vi "Add Message Handler.vi"(8 "error in (no error)":errorcluster, 10 "TCPMessageHandler":refnum<class "TCPMessageHandler.lvclass">, 11 "TCPMessaging in":refnum<class "TCPMessaging.lvclass">) -> (0 "error out":errorcluster, 3 "TCPMessaging out":refnum<class "TCPMessaging.lvclass">)   [LabVIEW 2020, in "Vecto.lvlib" / "TCPMessaging.lvclass"]
uses:
  TCPMessaging.lvclass
  TCPMessageHandler/TCPMessageHandler.lvclass
  TCPMessaging.lvclass/TCPMessaging.ctl
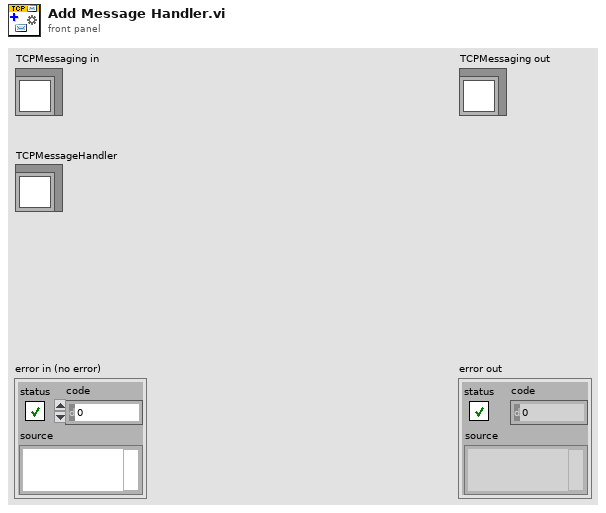
[diagram p1: front panel]
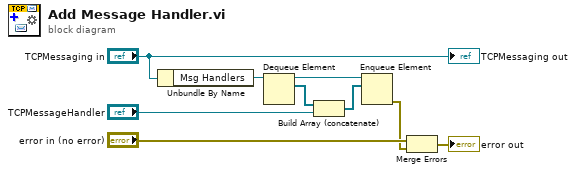
[diagram p0: block diagram]
diagram:
  n1 = Unbundle By Name("TCPMessaging in") -> ("Msg Handlers"=w8:refnum<queue>)
  n2 = Dequeue Element(queue=w8) -> (queue out=w5:refnum<queue>, element=w6:refnum<class "TCPMessageHandler.lvclass">[])  [unwired: 2 in, 2 out]
  n3 = Build Array (concatenate)(w6, "TCPMessageHandler") -> (w4:refnum<class "TCPMessageHandler.lvclass">[])
  n4 = Enqueue Element(queue=w5, element=w4) -> (error out=w1:errorcluster)  [unwired: 2 in, 2 out]
  n5 = Merge Errors("error in (no error)", w1) -> (→"error out":errorcluster)
  "TCPMessaging out" <- "TCPMessaging in"
